vi "Aurdino Mode Lights.vi"(0 "Climb":bool, 7 "Tracks Down":bool, 8 "Robot Centric":bool, 9 "Field Centric":bool) -> ()   [LabVIEW 2017]
uses:
  <vilib>/Rock Robotics/Network Tables/NT Read Boolean.vi
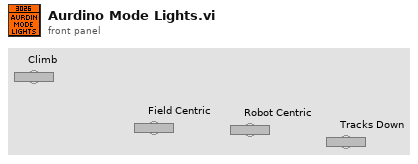
[diagram p1: front panel]
types:
  T1 = typedef "WPI_DigitalInputDevRef.ctl" = cluster{"DevStatus":errorcluster, "DIO Channel":T2}
  T2 = typedef "FPGA_DIOChannel.ctl" = enum8{"DIO 0", "DIO 1", "DIO 2", "DIO 3", "DIO 4", "DIO 5", "DIO 6", "DIO 7", "DIO 8", "DIO 9", "DIO MXP 0", "DIO MXP 1", "DIO MXP 2", "DIO MXP 3", "DIO MXP 4", "DIO MXP 5", "DIO MXP 6", "DIO MXP 7", "DIO MXP 8", "DIO MXP 9", "DIO MXP 10", "DIO MXP 11", "DIO MXP 12", "DIO MXP 13", "DIO MXP 14", "DIO MXP 15", "SPI Port CS1", "SPI Port CS2", "SPI Port CS3", "SPI Port MISO", "SPI Port MOSI", "Invalid"}
  T3 = typedef "WPI_DigitalOutputDevRef.ctl" = cluster{"DIO Channel":T2, "DevStatus":errorcluster}
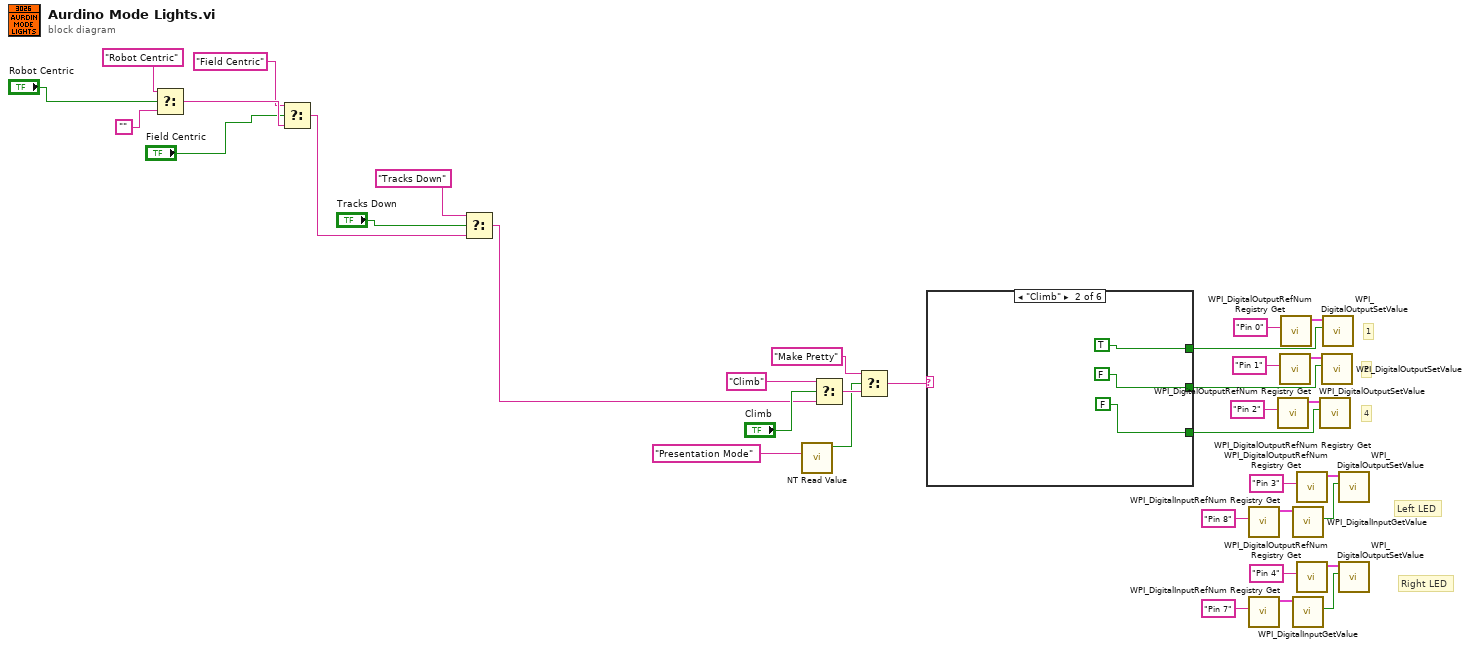
[diagram p0: block diagram]
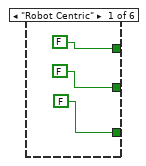
[diagram p2: hidden frame]
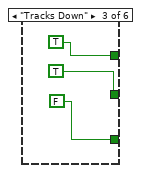
[diagram p3: hidden frame]
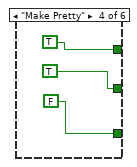
[diagram p4: hidden frame]
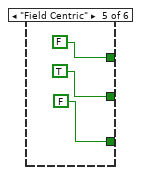
[diagram p5: hidden frame]
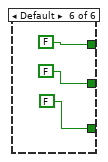
[diagram p6: hidden frame]
diagram:
  # "Right LED"
  # "Left LED"
  # "4"
  # "2"
  # "1"
  n1 = Select(t="Robot Centric", s="Robot Centric", f="") -> (s? t:f=w28:string)
  n2 = Select(t="Field Centric", s="Field Centric", f=w28) -> (s? t:f=w26:string)
  n3 = Select(t="Tracks Down", s="Tracks Down", f=w26) -> (s? t:f=w8:string)
  n4 = call-poly <vilib>:"NT Read Value.vi"("Name"="Presentation Mode") -> ("Boolean"=w2:bool)  [unwired: 9 in, 1 out]
  n5 = Select(t="Climb", s="Climb", f=w8) -> (s? t:f=w19:string)
  n6 = Select(t="Make Pretty", s=w2, f=w19) -> (s? t:f=w20:string)
  n7 = case shown="\"Climb\"" w20 {
    tunnel: [FALSE TRUE TRUE TRUE FALSE FALSE] -> w12
    tunnel: [FALSE FALSE TRUE TRUE TRUE FALSE] -> w13
    tunnel: [FALSE FALSE FALSE FALSE FALSE FALSE] -> w14
    frame "Robot Centric" {
    }
    frame "Climb" {
    }
    frame "Tracks Down" {
    }
    frame "Make Pretty" {
    }
    frame "Field Centric" {
    }
    frame Default {
    }
  }
  n8 = call <vilib>:"WPI_DigitalInputRefNum Registry Get.vi"("refnum name"="Pin 8") -> ("DigitalInputDevRef"=w17:T1)  [unwired: 9 in, 1 out]
  n9 = call <vilib>:"WPI_DigitalInputRefNum Registry Get.vi"("refnum name"="Pin 7") -> ("DigitalInputDevRef"=w7:T1)  [unwired: 9 in, 1 out]
  n10 = call <vilib>:"WPI_DigitalOutputRefNum Registry Get.vi"("refnum name"="Pin 2") -> ("DigitalOutputDevRef"=w34:T3)  [unwired: 9 in, 1 out]
  n11 = call <vilib>:"WPI_DigitalOutputRefNum Registry Get.vi"("refnum name"="Pin 1") -> ("DigitalOutputDevRef"=w35:T3)  [unwired: 9 in, 1 out]
  n12 = call <vilib>:"WPI_DigitalOutputRefNum Registry Get.vi"("refnum name"="Pin 0") -> ("DigitalOutputDevRef"=w36:T3)  [unwired: 9 in, 1 out]
  n13 = call <vilib>:"WPI_DigitalInputGetValue.vi"("DigitalInputDevRef"=w17) -> ("Value"=w11:bool)  [unwired: 8 in, 2 out]
  n14 = call <vilib>:"WPI_DigitalInputGetValue.vi"("DigitalInputDevRef"=w7) -> ("Value"=w4:bool)  [unwired: 8 in, 2 out]
  n15 = call <vilib>:"WPI_DigitalOutputRefNum Registry Get.vi"("refnum name"="Pin 3") -> ("DigitalOutputDevRef"=w33:T3)  [unwired: 9 in, 1 out]
  n16 = call <vilib>:"WPI_DigitalOutputRefNum Registry Get.vi"("refnum name"="Pin 4") -> ("DigitalOutputDevRef"=w5:T3)  [unwired: 9 in, 1 out]
  n17 = call <vilib>:"WPI_DigitalOutputSetValue.vi"("Value"=w14, "DigitalOutputDevRef"=w34) -> ()  [unwired: 8 in, 2 out]
  n18 = call <vilib>:"WPI_DigitalOutputSetValue.vi"("Value"=w13, "DigitalOutputDevRef"=w35) -> ()  [unwired: 8 in, 2 out]
  n19 = call <vilib>:"WPI_DigitalOutputSetValue.vi"("Value"=w12, "DigitalOutputDevRef"=w36) -> ()  [unwired: 8 in, 2 out]
  n20 = call <vilib>:"WPI_DigitalOutputSetValue.vi"("Value"=w11, "DigitalOutputDevRef"=w33) -> ()  [unwired: 8 in, 2 out]
  n21 = call <vilib>:"WPI_DigitalOutputSetValue.vi"("Value"=w4, "DigitalOutputDevRef"=w5) -> ()  [unwired: 8 in, 2 out]
